vi "InitMenu.vi"(8 "error in (no error)":errorcluster, 11 "Game in":refnum<class "Game.lvclass">) -> (0 "error out":errorcluster, 3 "Game out":refnum<class "Game.lvclass">)   [LabVIEW 2019, in "RT_Game.lvlib" / "Game.lvclass"]
uses:
  Game.lvclass
  GameMenu/GameMenu.lvclass
  GameMenu/GameMenu.lvclass/GameMenu.ctl
  Game.lvclass/Game.ctl
  GameMenu/Write Active_.vi
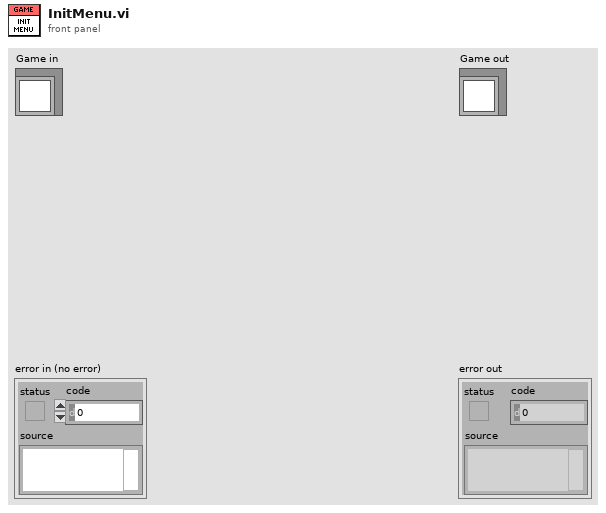
[diagram p1: front panel]
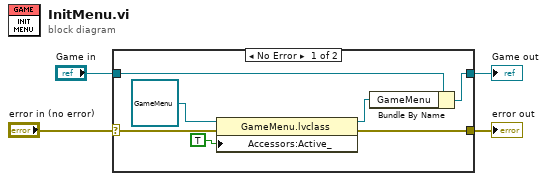
[diagram p0: block diagram]
diagram:
  n1 = case shown="No Error" "error in (no error)" {
    selector: "error in (no error)" -> [w10 w13]
    tunnel: [w8 w13] -> w3
    tunnel: [w9 w12] -> w1
    tunnel: "Game in" -> [w11 w12]
    frame No Error {
      n2 = property class="GameMenu.lvclass"(reference=refnum<class "GameMenu.lvclass"> refnum ("GameMenu"), error in=w10, "Accessors:Active_"=TRUE ("Active_")) -> (reference out=w6:refnum<class "GameMenu.lvclass">, error out=w8:errorcluster)
      n3 = Bundle By Name(cluster=w11, "GameMenu"=w6) -> (w9:refnum<class "Game.lvclass">)
    }
    frame Error {
    }
  }
  "error out" <- w3
  "Game out" <- w1
